vi "InputCurve.vi"(10 "Throttle Cluster":T1={"Neutral Signal"=512.0, "Bottom Deadzone"=707.070707070707, "Neutral Deadzone"=0.0, "Top Cutout"=971.4285714285714, "Bottom Cutout"=89.79591836734694, "Top Deadzone"=64627.90909090909, "Throttle Curve Type"=enum."Linear"} {"Top Deadzone" scale=55537.0..65537.0; "Bottom Cutout" scale=0.0..200.0; "Top Cutout" scale=800.0..1024.0; "Neutral Deadzone" scale=0.0..10000.0; "Bottom Deadzone" scale=1.0..10000.0; "Neutral Signal" scale=480.0..544.0}, 11 "Input":i32) -> (2 "Output":dbl, 3 "Throttle Graph":cluster{dbl[], dbl[]}[](graph))   [LabVIEW 2013]
panel:
  out "Raw":i32
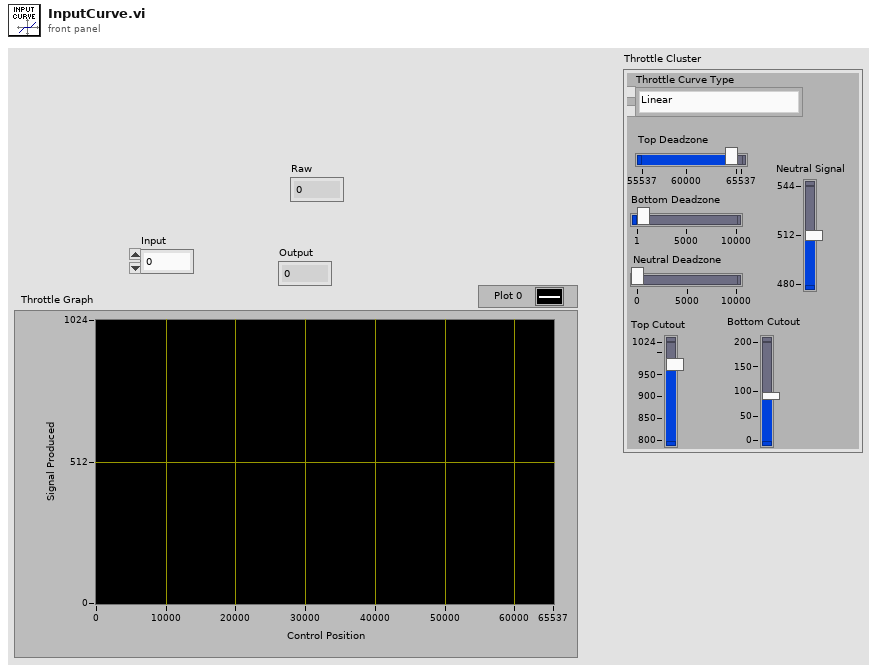
[diagram p1: front panel]
types:
  T1 = cluster{"Neutral Signal":dbl, "Bottom Deadzone":dbl, "Neutral Deadzone":dbl, "Top Cutout":dbl, "Bottom Cutout":dbl, "Top Deadzone":dbl, "Throttle Curve Type":enum16{"Linear", "Linear, No Deadzone", "Logarithmic", "Exponental"}}
  T2 = enum16{"Linear", "Linear, No Deadzone", "Logarithmic", "Exponental"}
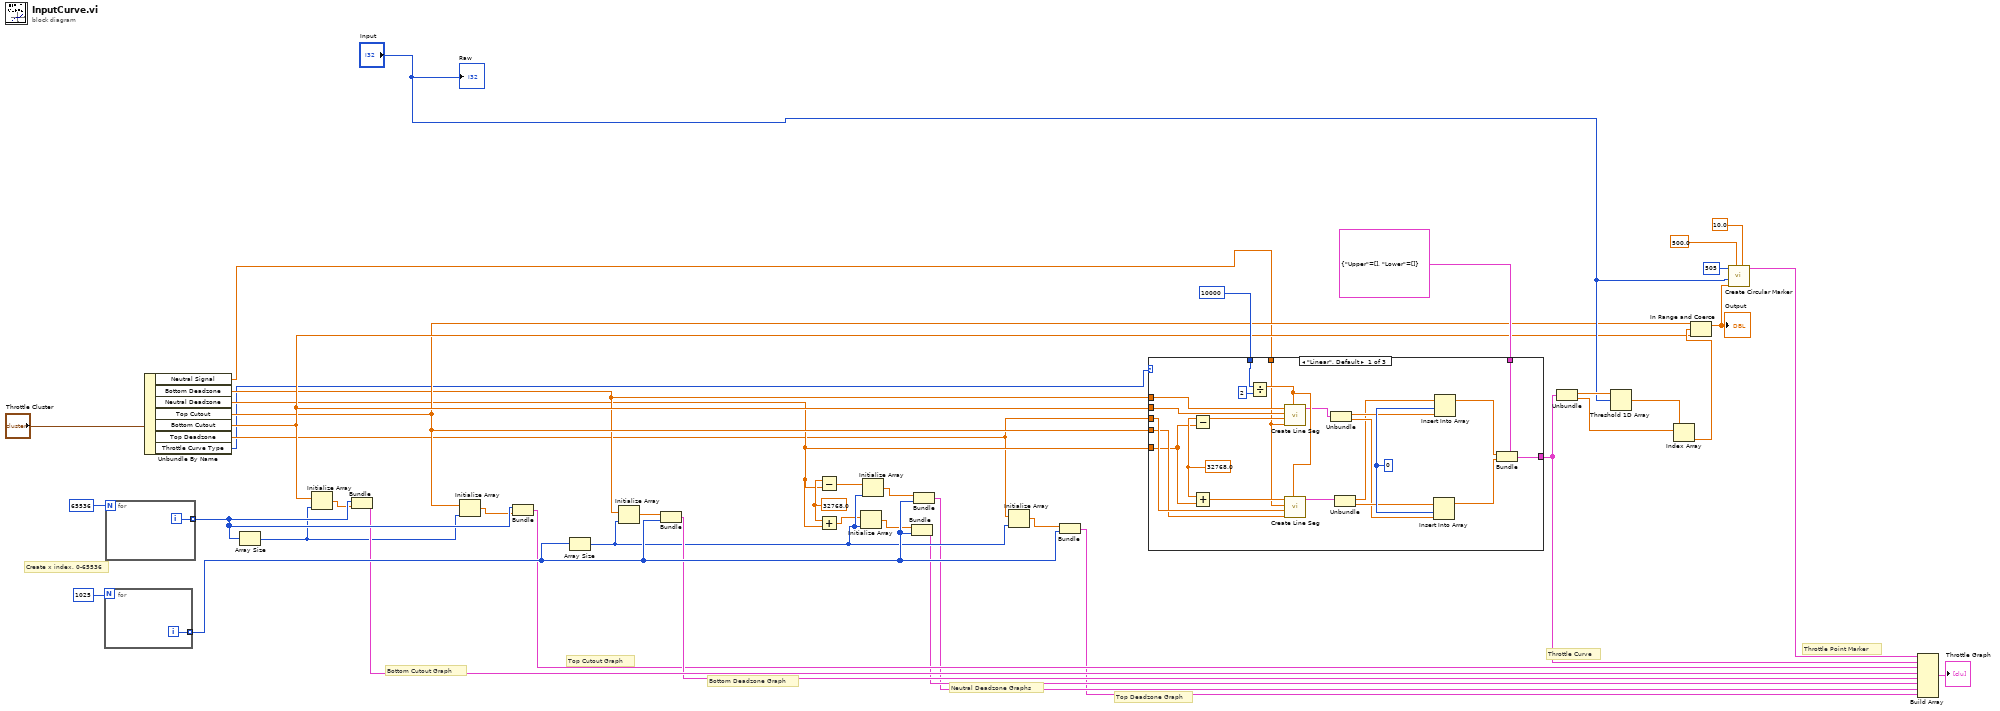
[diagram p0: block diagram]
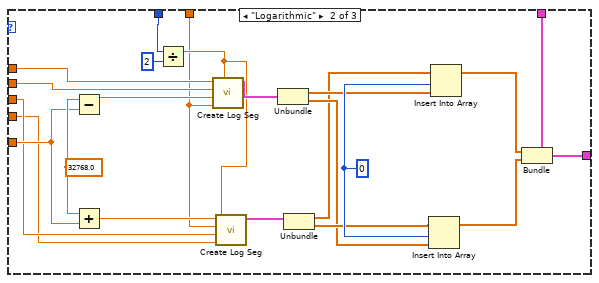
[diagram p2: hidden frame]
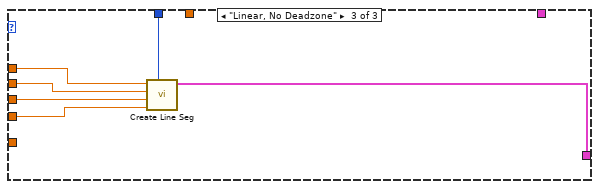
[diagram p3: hidden frame]
diagram:
  w26 = 32768.0 ("y")
  # "Neutral Deadzone Graphs"
  # "Throttle Point Marker"
  # "Top Deadzone Graph"
  # "Bottom Deadzone Graph"
  # "Bottom Cutout Graph"
  # "Throttle Curve"
  # "Top Cutout Graph"
  # "Create x index, 0-65536"
  n1 = for {
    N: 1025 -> [_]
    tunnel: [w44] -> w41 mode=indexing
    i -> [w44]
  }
  n2 = for {
    N: 65536 -> [_]
    tunnel: [w45] -> w43 mode=indexing
    i -> [w45]
  }
  n3 = Unbundle By Name("Throttle Cluster") -> ("Neutral Signal"=w1:dbl, "Bottom Deadzone"=w5:dbl, "Neutral Deadzone"=w4:dbl, "Top Cutout"=w6:dbl, "Bottom Cutout"=w7:dbl, "Top Deadzone"=w3:dbl, "Throttle Curve Type"=w2:T2)
  n4 = Array Size(array=w43) -> (size(s)=w32:i32)
  n5 = Initialize Array(w7, w32) -> (w37:dbl[])
  n6 = Bundle(w43, w37) -> (w36:cluster{i32[], dbl[]})  [unwired: 1 in]
  n7 = Initialize Array(w6, w32) -> (w38:dbl[])
  n8 = Bundle(w43, w38) -> (w31:cluster{i32[], dbl[]})  [unwired: 1 in]
  n9 = Array Size(array=w41) -> (size(s)=w23:i32)
  n10 = Initialize Array(w5, w23) -> (w35:dbl[])
  n11 = Bundle(w35, w41) -> (w33:cluster{dbl[], i32[]})  [unwired: 1 in]
  n12 = Subtract(x=w26, y=w4) -> (x-y=w21:dbl)
  n13 = Add(x=w26, y=w4) -> (x+y=w22:dbl)
  n14 = Initialize Array(w22, w23) -> (w24:dbl[])
  n15 = Initialize Array(w21, w23) -> (w25:dbl[])
  n16 = Bundle(w24, w41) -> (w20:cluster{dbl[], i32[]})  [unwired: 1 in]
  n17 = Bundle(w25, w41) -> (w19:cluster{dbl[], i32[]})  [unwired: 1 in]
  n18 = Initialize Array(w3, w23) -> (w34:dbl[])
  n19 = Bundle(w34, w41) -> (w18:cluster{dbl[], i32[]})  [unwired: 1 in]
  n20 = case shown="\"Linear\", Default" w2 {
    tunnel: w7 -> [w68 w78 w97]
    tunnel: w6 -> [w64 w71 w96]
    tunnel: w5 -> [w67 w77 w95]
    tunnel: w3 -> [w65 w72 w94]
    tunnel: [w55 w87 w93] -> w29
    tunnel: w4 -> [w53 w85 _]
    tunnel: 10000 ("Number of Points") -> [w52 w84 w92]
    tunnel: w1 -> [w47 w73 _]
    tunnel: cluster{"Upper":dbl[], "Lower":dbl[]} {"Upper"=[], "Lower"=[]} -> [w46 w69 _]
    frame "Linear", Default {
      w58 = 0 ("index")
      w54 = 32768.0 ("y")
      n21 = Subtract(x=w54, y=w53) -> (x-y=w66:dbl)
      n22 = Add(x=w54, y=w53) -> (x+y=w63:dbl)
      n23 = Divide(x=w52, y=2) -> (x/y=w61:dbl)
      n24 = call "Create Line Seg.vi"("Number of Points"=w61, "Y 2"=w47, "X 2"=w66, "Y 1"=w68, "X 1"=w67) -> ("Line Segment"=w60:cluster{dbl[], dbl[]})  [unwired: 5 in]
      n25 = call "Create Line Seg.vi"("Number of Points"=w61, "Y 2"=w64, "X 2"=w65, "Y 1"=w47, "X 1"=w63) -> ("Line Segment"=w59:cluster{dbl[], dbl[]})  [unwired: 5 in]
      n26 = Unbundle(w60) -> (w49:dbl[], w50:dbl[])
      n27 = Unbundle(w59) -> (w48:dbl[], w51:dbl[])
      n28 = Insert Into Array(array=w51, index=w58, new element=w50) -> (w56:dbl[])
      n29 = Insert Into Array(array=w48, index=w58, new element=w49) -> (w57:dbl[])
      n30 = Bundle(cluster=w46, "Upper"=w57, "Lower"=w56) -> (w55:cluster{"Upper":dbl[], "Lower":dbl[]})
    }
    frame "Logarithmic" {
      w90 = 0 ("index")
      w86 = 32768.0 ("y")
      n31 = Subtract(x=w86, y=w85) -> (x-y=w79:dbl)
      n32 = Add(x=w86, y=w85) -> (x+y=w74:dbl)
      n33 = Divide(x=w84, y=2) -> (x/y=w75:dbl)
      n34 = call "Create Log Seg.vi"("Number of Points"=w75, "Y 2"=w73, "X 2"=w79, "Y 1"=w78, "X 1"=w77) -> ("Line Segment"=w76:cluster{dbl[], dbl[]})  [unwired: 5 in]
      n35 = call "Create Log Seg.vi"("Number of Points"=w75, "Y 2"=w71, "X 2"=w72, "Y 1"=w73, "X 1"=w74) -> ("Line Segment"=w70:cluster{dbl[], dbl[]})  [unwired: 5 in]
      n36 = Unbundle(w76) -> (w81:dbl[], w82:dbl[])
      n37 = Unbundle(w70) -> (w80:dbl[], w83:dbl[])
      n38 = Insert Into Array(array=w83, index=w90, new element=w82) -> (w88:dbl[])
      n39 = Insert Into Array(array=w80, index=w90, new element=w81) -> (w89:dbl[])
      n40 = Bundle(cluster=w69, "Upper"=w89, "Lower"=w88) -> (w87:cluster{"Upper":dbl[], "Lower":dbl[]})
    }
    frame "Linear, No Deadzone" {
      n41 = call "Create Line Seg.vi"("Number of Points"=w92, "Y 2"=w96, "X 2"=w94, "Y 1"=w97, "X 1"=w95) -> ("Line Segment"=w93:cluster{dbl[], dbl[]})  [unwired: 5 in]
    }
  }
  n42 = Unbundle(w29) -> ("Upper"=w13:dbl[], "Lower"=w15:dbl[])
  n43 = Threshold 1D Array(2:"Input", 3:w13) -> (0:w14:dbl)  [unwired: 1 in]
  n44 = Index Array(array=w15, index=w14) -> (element=w30:dbl)
  n45 = In Range and Coerce(upper limit=w6, x=w30, lower limit=w7) -> (coerced(x)=w11:dbl)  [unwired: 1 out]
  "Output" <- w11
  n46 = call "Create Circular Marker.vi"("Y Radius"=10.0, "X Radius"=500.0, "Y Center"=w11, "X Center"="Input", "Number of Points"=505) -> ("XY Graph"=w28:cluster{dbl[], dbl[]})  [unwired: 6 in]
  n47 = Build Array(w28, w29, w31, w36, w33, w20, w19, w18) -> (→"Throttle Graph":cluster{"Upper":dbl[], "Lower":dbl[]}[])
  "Raw" <- "Input"
